vi "GetFlatSequences.vi"(6 "error in":errorcluster, 9 "VI Interpreter in":refnum<class "VI Interpreter.lvclass">) -> (0 "error out":errorcluster, 3 "VI Interpreter out":refnum<class "VI Interpreter.lvclass">)   [LabVIEW 2014, in "VI Interpreter.lvclass"]
uses:
  VI Interpreter.lvclass
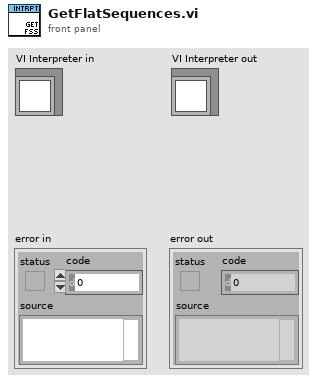
[diagram p1: front panel]
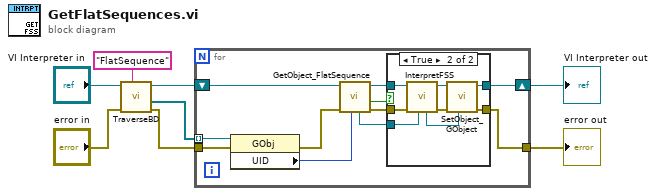
[diagram p0: block diagram]
diagram:
  n1 = call "TraverseBD.vi"("class name"="FlatSequence", "error in"="error in", "VI Interpreter in"="VI Interpreter in") -> ("error out"=w4:errorcluster, "References"=w2:refnum<vi>[], "VI Interpreter out"=w5:refnum<class "VI Interpreter.lvclass">)  [unwired: 4 in]
  n2 = for {
    tunnel: w2 -> [w18] mode=indexing
    shift-right: [w12] -> w8
    shift-left: w5 -> [w19]
    tunnel: w4 -> [w17]
    tunnel: [w11] -> w7
    n3 = property class="GObj"(reference=w18, error in=w17) -> (error out=w16:errorcluster, "UID"=w9:i32)  [unwired: 1 out]
    n4 = call "GetObject_FlatSequence.vi"("UID"=w9, "error in"=w16, "VI Interpreter in"=w19) -> ("error out"=w13:errorcluster, "found"=w10:bool, "VI Interpreter out"=w15:refnum<class "VI Interpreter.lvclass">, "flat sequence"=w14:refnum<class "FlatSequence.lvclass">)  [unwired: 3 in]
    n5 = case shown="True" w10 {
      tunnel: w15 -> [w21 w27]
      tunnel: w14 -> [_ w23]
      tunnel: w13 -> [w20 w25]
      tunnel: [w21 w29] -> w12
      tunnel: [w20 w28] -> w11
      frame False {
      }
      frame True {
        n6 = call "InterpretFSS.vi"("FSS in"=w23, "error in"=w25, "VI Interpreter in"=w27) -> ("error out"=w24:errorcluster, "VI Interpreter out"=w26:refnum<class "VI Interpreter.lvclass">, "FSS out"=w22:refnum<class "FlatSequence.lvclass">)  [unwired: 4 in]
        n7 = call "SetObject_GObject.vi"("GObject"=w22, "error in"=w24, "VI Interpreter in"=w26) -> ("error out"=w28:errorcluster, "VI Interpreter out"=w29:refnum<class "VI Interpreter.lvclass">)  [unwired: 5 in]
      }
    }
  }
  "error out" <- w7
  "VI Interpreter out" <- w8
